vi "MU Calibration set Current Analog Track Adjustments.vi"(8 "error in (no error)":errorcluster, 9 "noniusAdjustments":T1, 10 "masterAdjustments":T1, 11 "CalibrationHandle":T2) -> (0 "error out":errorcluster, 3 "function return":bool)   [LabVIEW 2017, in "MU_3SL_interface.lvlib"]
doc: "MU_PUBLIC bool MU_Calibration_setCurrentAnalogTrackAdjustments(\n MU_Calibration* calibration,\n const MU_Calibration_AnalogTrackAdjustments* masterAdjustments,\n const MU_Calibration_AnalogTrackAdjustments* noniusAdjustments);"
uses:
  MU_3SL_interface.lvlib
  handles/CalibrationHandle.ctl
  lib/MU_3SL_interface.dll
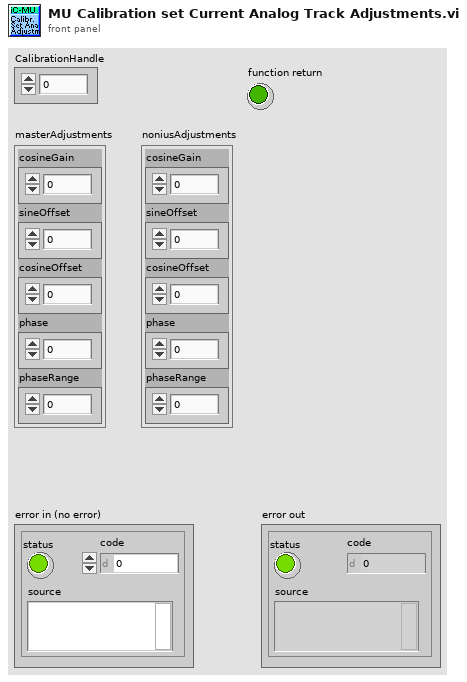
[diagram p1: front panel]
types:
  T1 = cluster{"cosineGain":u8, "sineOffset":u8, "cosineOffset":u8, "phase":u8, "phaseRange":u8}
  T2 = typedef "MU_3SL_interface.lvlib/CalibrationHandle.ctl" = u64
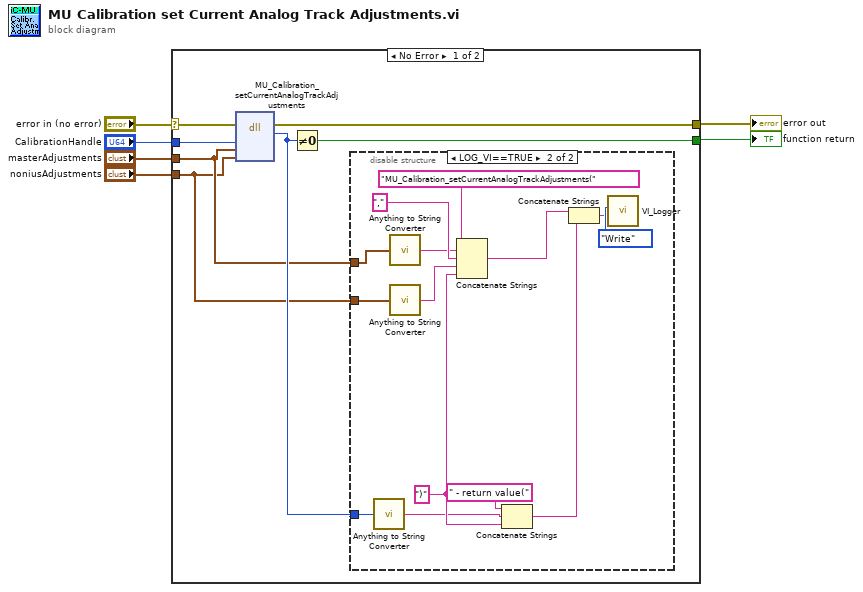
[diagram p0: block diagram]
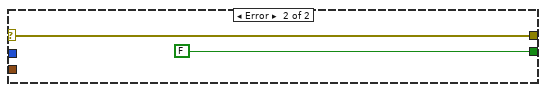
[diagram p3: hidden frame]
diagram:
  n1 = case shown="No Error" "error in (no error)" {
    selector: "error in (no error)" -> [w11 w28]
    tunnel: [w13 FALSE] -> w6
    tunnel: "masterAdjustments" -> [w9 _]
    tunnel: "noniusAdjustments" -> [w8 _]
    tunnel: [w7 w28] -> w4
    tunnel: "CalibrationHandle" -> [w12 _]
    frame No Error {
      n2 = dll-call lib="C:/Users/bes/AppData/Roaming/work/mu_9so/icsubmodules/soft_mu_3sl_master/lv_interface/lib/MU_3SL_interface**.*" fn="MU_Calibration_setCurrentAnalogTrackAdjustments"(error in=w11, "CalibrationHandle"=w12, "masterAdjustments"=w9, "noniusAdjustments"=w8) -> (error out=w7:errorcluster, "return type"=w10:u8)  [unwired: 5 in, 1 out]
      n3 = Not Equal To 0?(x=w10) -> (x != 0?=w13:bool)
      n4 = disable-structure shown="LOG_VI==TRUE" {
        disable-tunnel: w10 -> [_ w16]
        disable-tunnel: w9 -> [_ w20]
        disable-tunnel: w8 -> [_ w18]
        frame condition #0 {
        }
        frame condition #1 (active) {
          w21 = ")" ("string")
          n5 = call "Anything to String Converter.vi"("anything"=w16) -> ("String"=w15:string)
          n6 = call "Anything to String Converter.vi"("anything"=w20) -> ("String"=w19:string)
          n7 = call "Anything to String Converter.vi"("anything"=w18) -> ("String"=w17:string)
          n8 = Concatenate Strings("MU_Calibration_setCurrentAnalogTrackAdjustments(" ("Info in"), w19, "," ("string"), w17, w21) -> (w14:string)
          n9 = Concatenate Strings(" - return value(" ("string"), w15, w21) -> (w25:string)
          n10 = Concatenate Strings(w14, w25) -> (w24:string)
          n11 = call "VI_Logger.vi"("Action (Read)"=enum16{"Write", "Read"}."Write", "Info in"=w24) -> ()  [unwired: 8 in, 2 out]
        }
      }
    }
    frame Error {
    }
  }
  "function return" <- w6
  "error out" <- w4
